vi "getNinePixelfromMemroy(n+1).vi"(0 "col":u16, 5 "row":u16, 7 "Width":u16, 9 "Memory In":refnum<k21>, 11 "divider":u8) -> (1 "1":i8, 2 "2":i8, 3 "3":i8, 4 "4":i8, 8 "5":i8, 12 "9":i8, 13 "8":i8, 14 "7":i8, 15 "6":i8)   [LabVIEW 2016]
uses:
  <vilib>/rvi/DataTransferAndStorage/Container/Common/niFpgaContainerExecOnDevCompGetState.vi
  <vilib>/rvi/Emulation/niFpgaEmulationIsFPGAContextNoSignature.vi
  <vilib>/rvi/DataTransferAndStorage/Container/Common/niFpgaContainerGetUniqueNameForEmu.vi
  <vilib>/rvi/Emulation/niFpgaProcessEmulError.vi
  <vilib>/rvi/Emulation/niFpgaSctlEmulationGetInTimedLoop.vi
  <vilib>/rvi/errors/nirviReportUnexpectedCaseInternalError (U32).vi
  <vilib>/rvi/Memory/Memory_Emulation/niFpgaMemoryEmulationCacheClearOnFirstRun.vi
  <vilib>/rvi/Memory/Memory_Emulation/nirvimemoryEmulationManagerCache_MakeExclusive.vi
  <vilib>/rvi/Memory/Memory_Emulation/niFpgaMemoryEmulationValidateCache.vi
  <vilib>/rvi/Memory/Memory_Emulation/nirvimemoryEmulationManagerCache_InsertValue.vi
  <vilib>/Utility/error.llb/Clear Errors.vi
  <vilib>/rvi/Memory/Memory_Emulation/nirvimemoryEmulationManagerCache_ReleaseExclusive.vi
  <vilib>/rvi/Memory/Memory_Emulation/nirvimemoryEmulationManagerCache_GetValue.vi
  <vilib>/rvi/Memory/Memory_Emulation/nirvimemoryEmulationManagerCache_SetValue.vi
  <vilib>/rvi/Emulation/niFpgaSctlEmulationResourceMgr.vi
  <vilib>/rvi/DataTransferAndStorage/Container/XNode/niFpgaContainer.xnode
  <vilib>/rvi/Memory/Memory_Emulation/niFpgaMemoryEmulationRefIn.vi
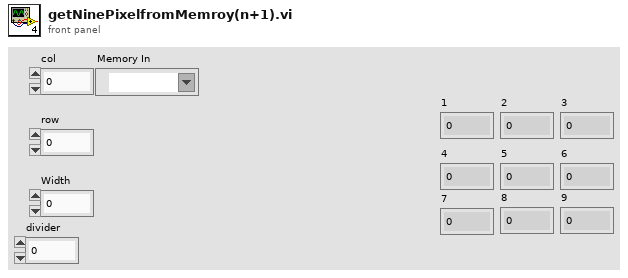
[diagram p1: front panel]
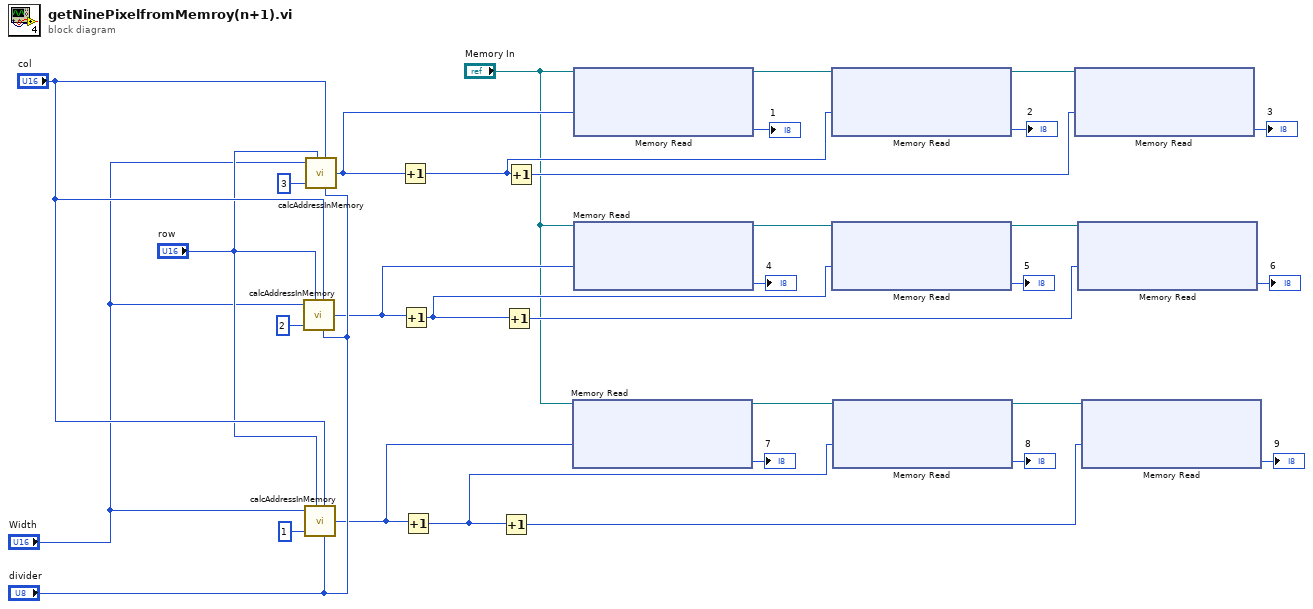
[diagram p0: block diagram]
diagram:
  n1 = call "calcAddressInMemory.vi"("Width"="Width", "Rows"="row", "delayRowCount"=u16 2, "Cols"="col", "divider"="divider") -> ("addressInMemory"=w18:u16)  [unwired: 4 in]
  n2 = call "calcAddressInMemory.vi"("Width"="Width", "Rows"="row", "delayRowCount"=u16 1, "Cols"="col", "divider"="divider") -> ("addressInMemory"=w12:u16)  [unwired: 4 in]
  n3 = call "calcAddressInMemory.vi"("Width"="Width", "Rows"="row", "delayRowCount"=u16 3, "Cols"="col", "divider"="divider") -> ("addressInMemory"=w25:u16)  [unwired: 4 in]
  n4 = Increment(x=w25) -> (x+1=w23:u16)
  n5 = Increment(x=w18) -> (x+1=w17:u16)
  n6 = Increment(x=w12) -> (x+1=w10:u16)
  n7 = Increment(x=w10) -> (x+1=w11:u16)
  n8 = Increment(x=w17) -> (x+1=w16:u16)
  n9 = Increment(x=w23) -> (x+1=w21:u16)
  n10 = xnode "Memory Read"("Address"=w12, "Memory In"="Memory In") -> ("Data"=→"7":i8, "Memory Out"=w15:refnum<k21>)
  n11 = xnode "Memory Read"("Address"=w25, "Memory In"="Memory In") -> ("Data"=→"1":i8, "Memory Out"=w24:refnum<k21>)
  n12 = xnode "Memory Read"("Address"=w18, "Memory In"="Memory In") -> ("Data"=→"4":i8, "Memory Out"=w19:refnum<k21>)
  n13 = xnode "Memory Read"("Address"=w23, "Memory In"=w24) -> ("Data"=→"2":i8, "Memory Out"=w22:refnum<k21>)
  n14 = xnode "Memory Read"("Address"=w17, "Memory In"=w19) -> ("Data"=→"5":i8, "Memory Out"=w20:refnum<k21>)
  n15 = xnode "Memory Read"("Address"=w10, "Memory In"=w15) -> ("Data"=→"8":i8, "Memory Out"=w14:refnum<k21>)
  n16 = xnode "Memory Read"("Address"=w21, "Memory In"=w22) -> ("Data"=→"3":i8)  [unwired: 1 out]
  n17 = xnode "Memory Read"("Address"=w16, "Memory In"=w20) -> ("Data"=→"6":i8)  [unwired: 1 out]
  n18 = xnode "Memory Read"("Address"=w11, "Memory In"=w14) -> ("Data"=→"9":i8)  [unwired: 1 out]
